vi "autonSample.vi"(0 "Auton Array":dbl[][](array[numeric]), 5 "MeasuredHeading":dbl, 9 "EncoderDistance":dbl) -> (4 "Left Drive":dbl(knob) scale=-1.0..1.0, 6 "Right Drive":dbl(knob) scale=-1.0..1.0, 10 "Turret Rotation":dbl, 14 "Feeder motor":dbl, 15 "Shooter motor output":dbl)   [LabVIEW 2011]
uses:
  Robot Global Data.vi
panel:
  out "Tzero":i64
  out "AccumDist":dbl
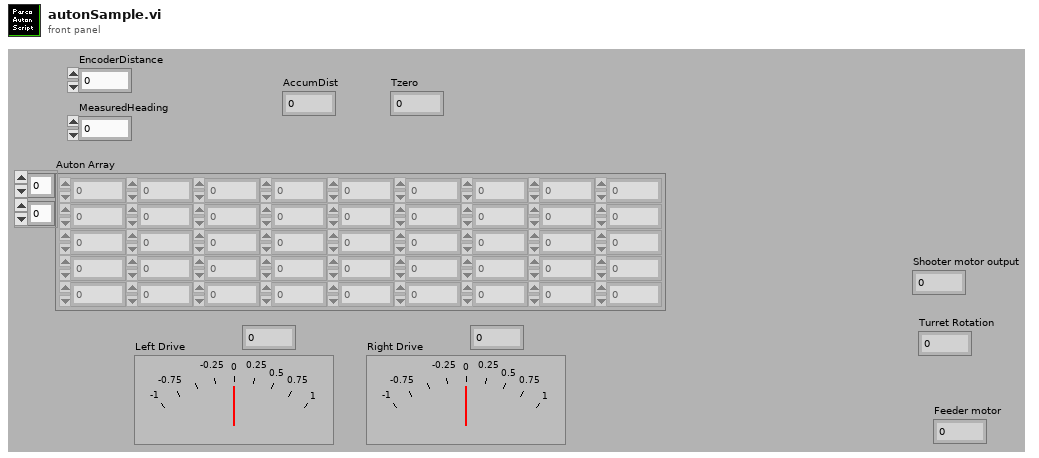
[diagram p1: front panel]
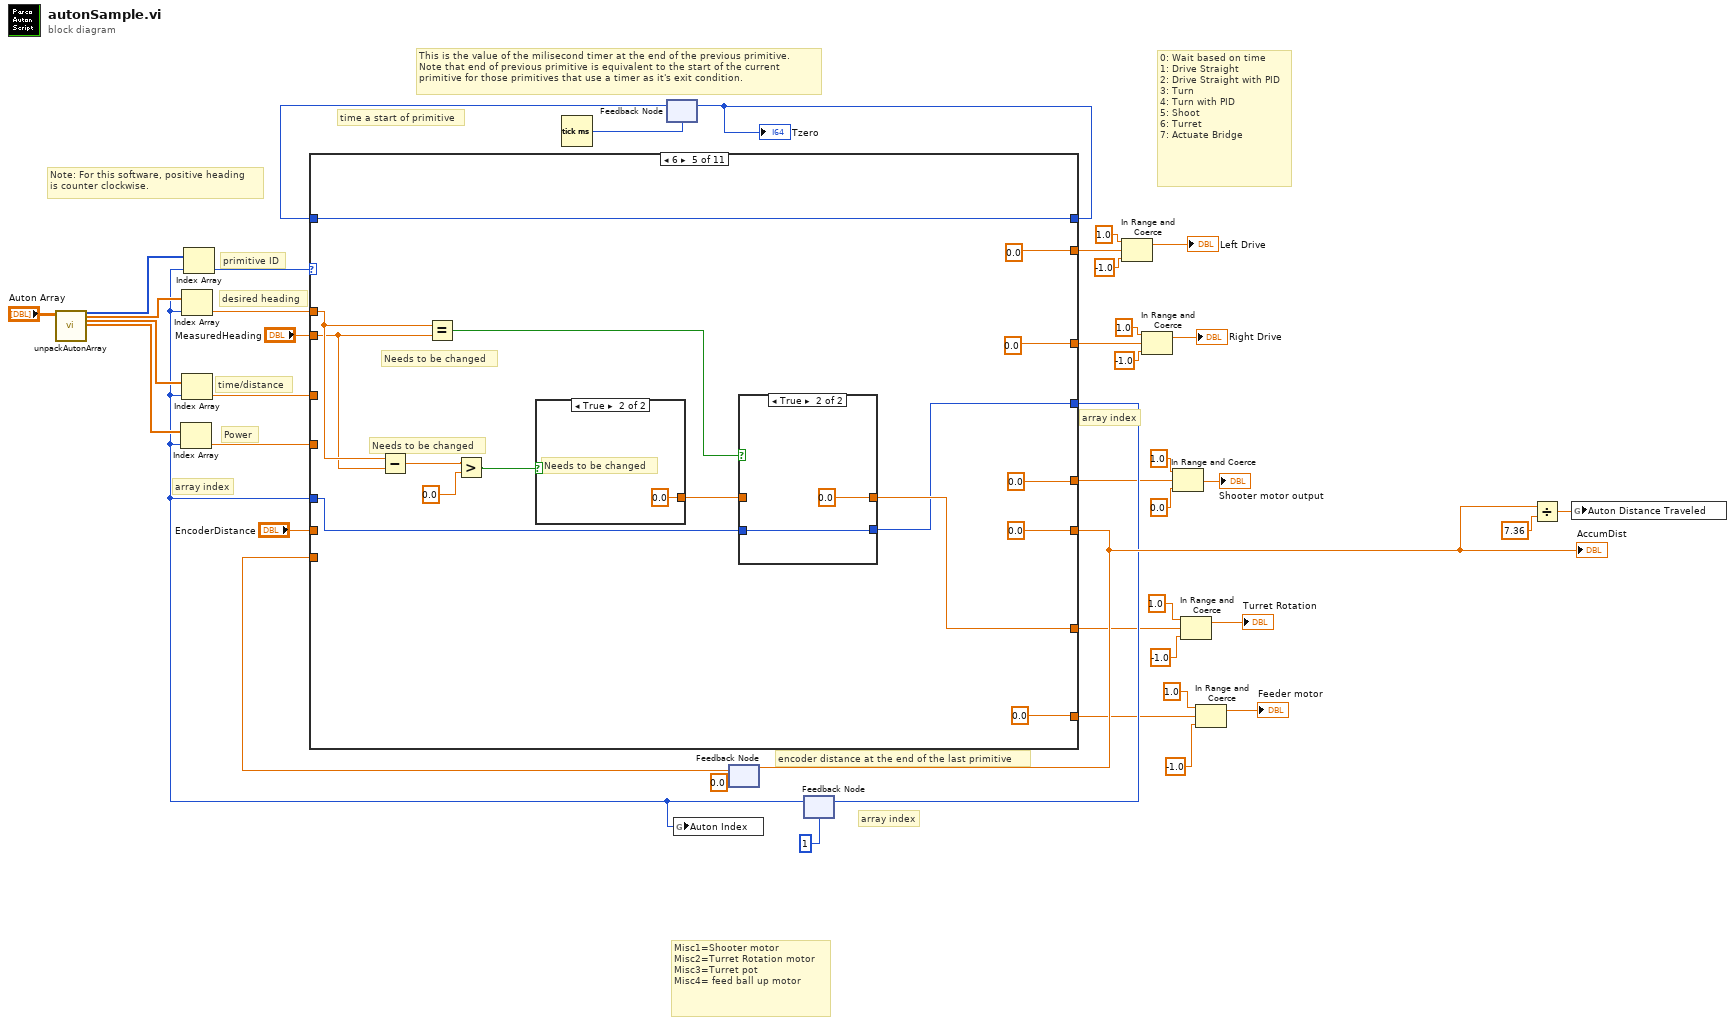
[diagram p0: block diagram]
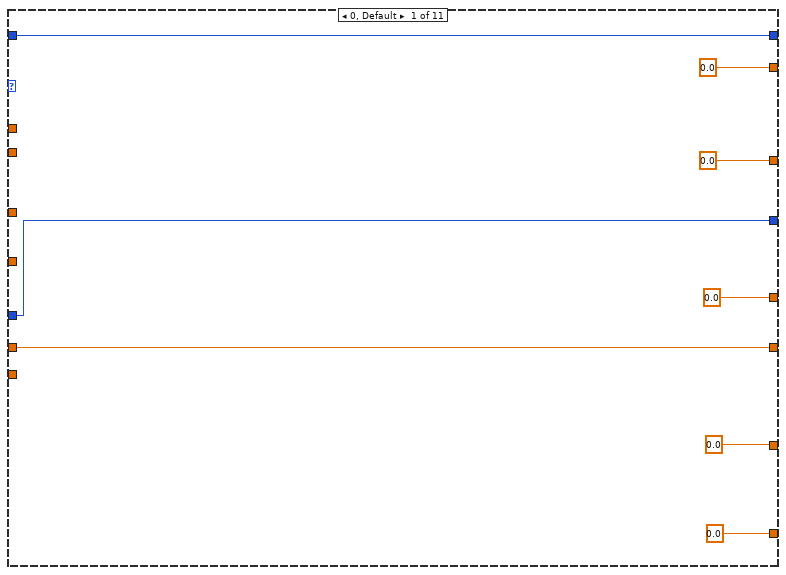
[diagram p2: hidden frame]
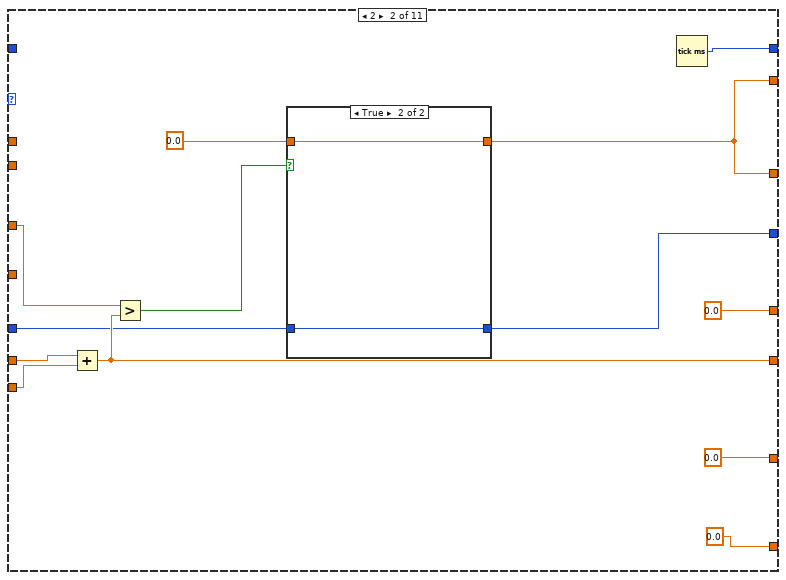
[diagram p3: hidden frame]
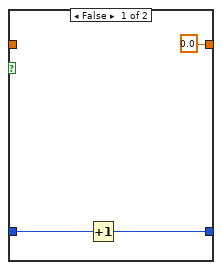
[diagram p4: hidden frame]
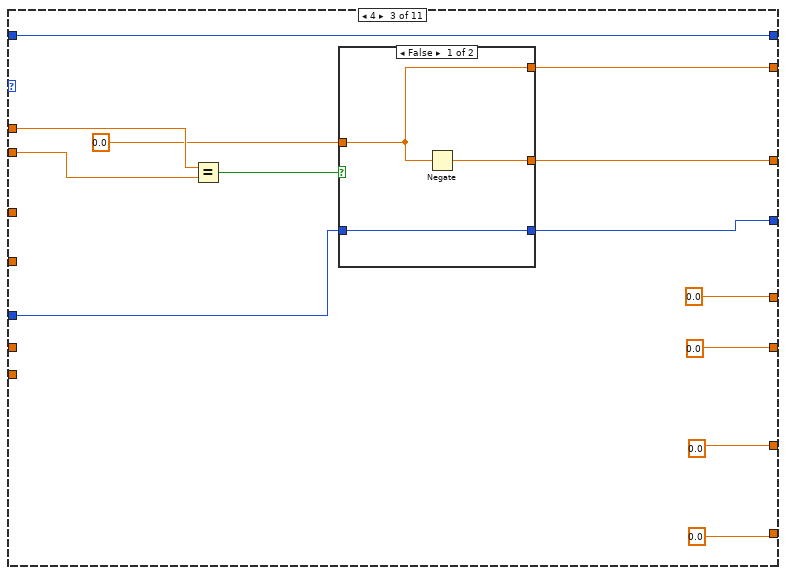
[diagram p5: hidden frame]
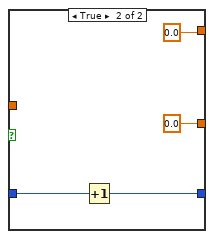
[diagram p6: hidden frame]
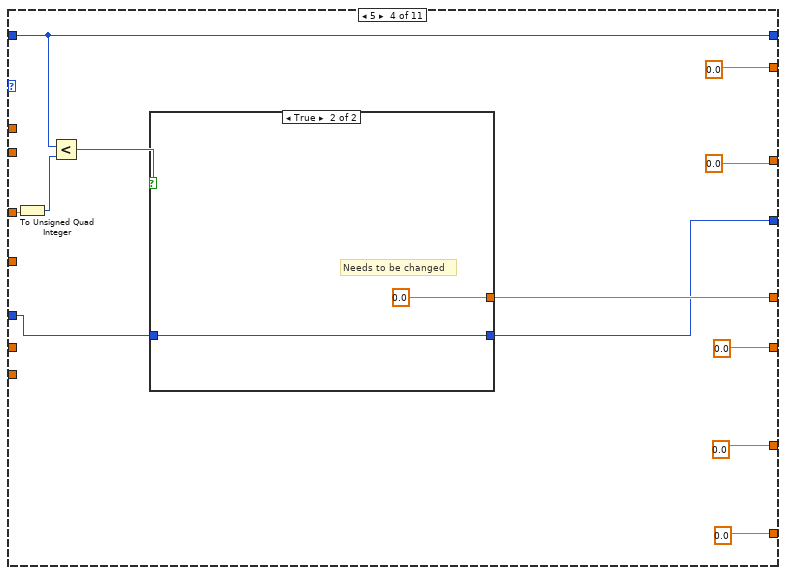
[diagram p7: hidden frame]
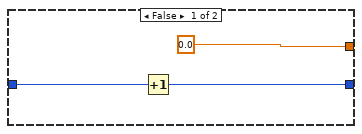
[diagram p8: hidden frame]
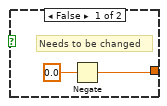
[diagram p10: hidden frame]
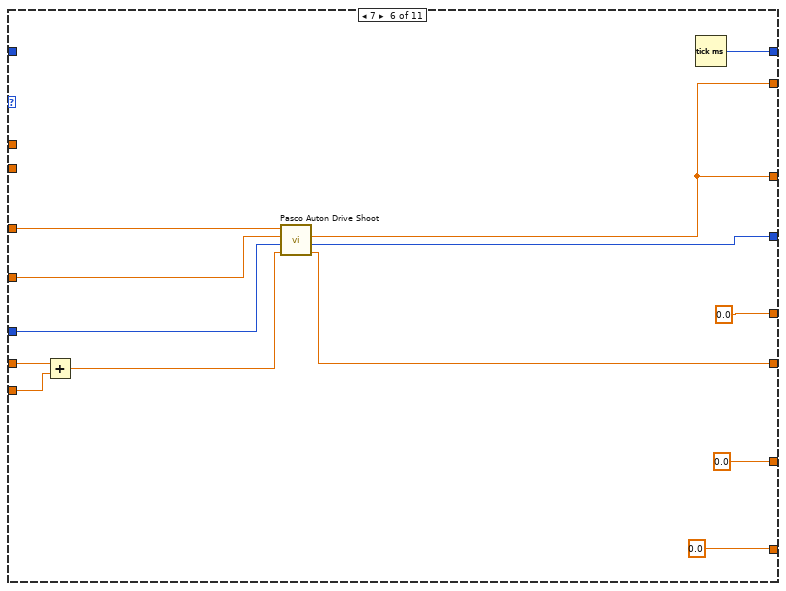
[diagram p11: hidden frame]
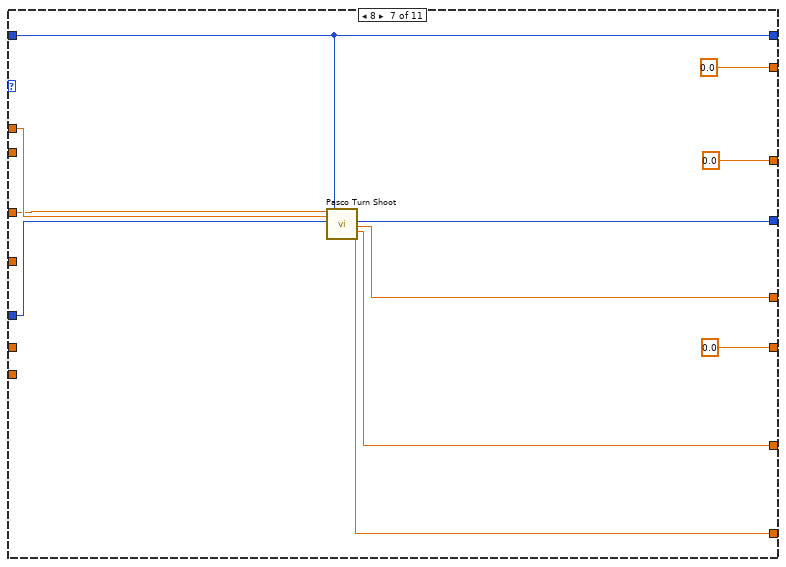
[diagram p12: hidden frame]
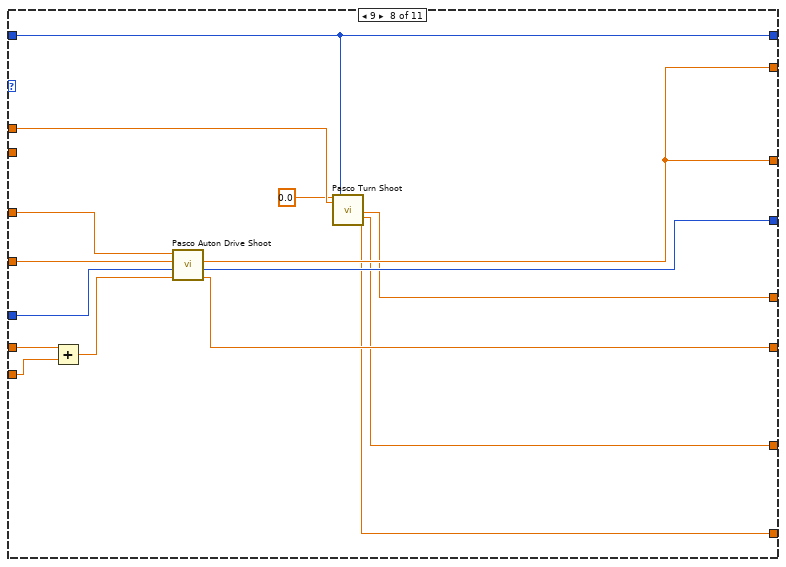
[diagram p13: hidden frame]
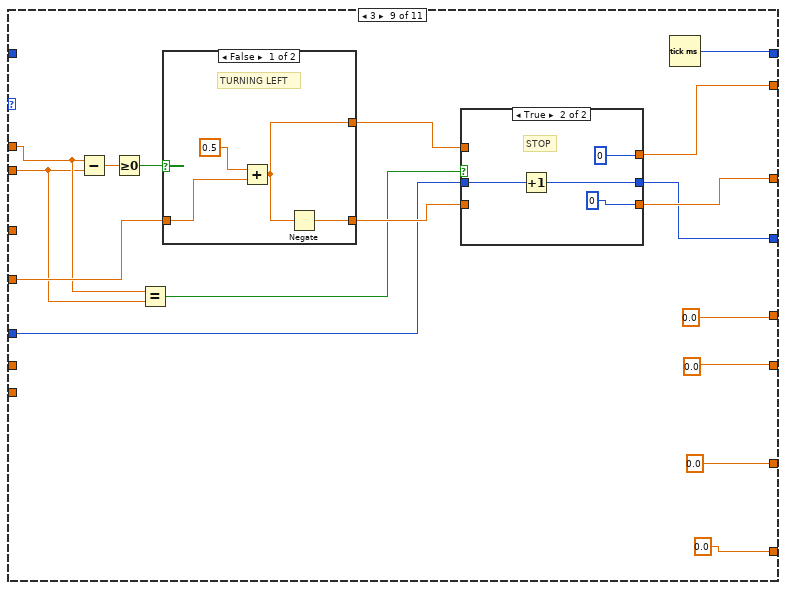
[diagram p14: hidden frame]
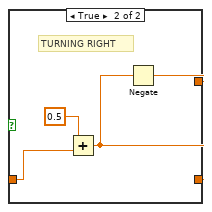
[diagram p16: hidden frame]
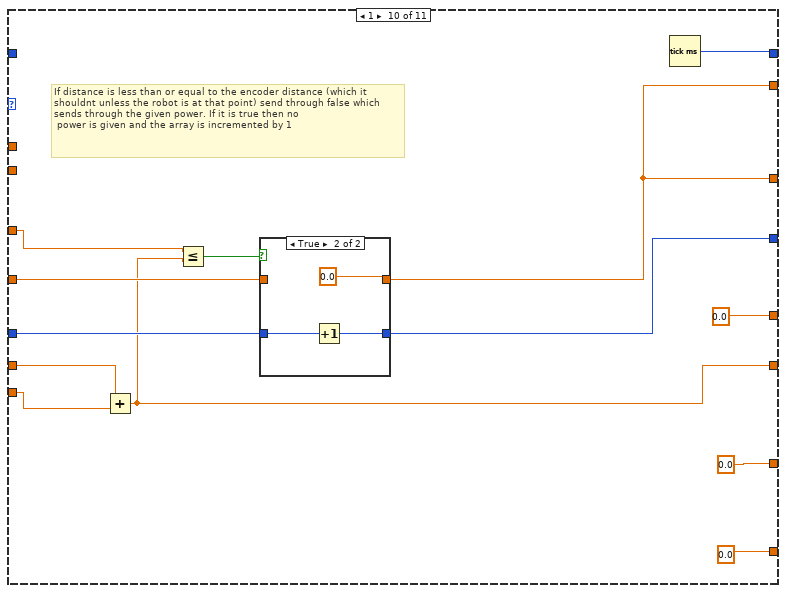
[diagram p17: hidden frame]
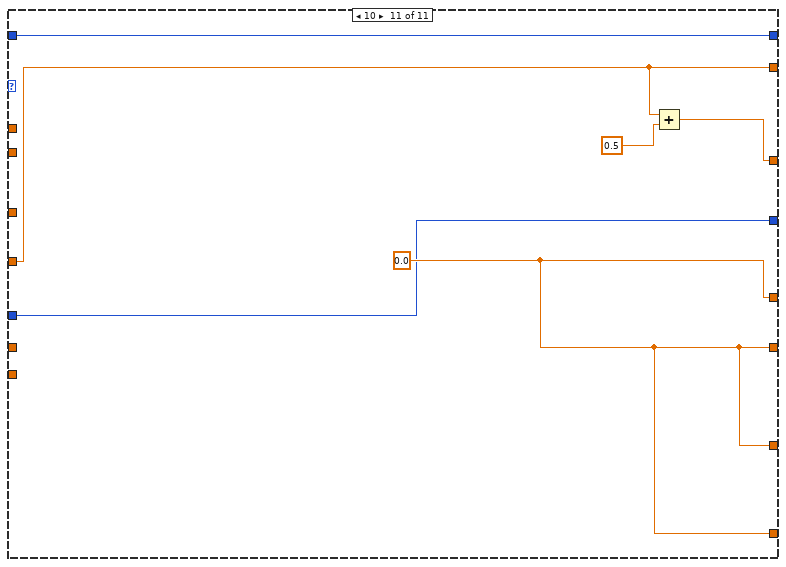
[diagram p19: hidden frame]
diagram:
  # "Misc1=Shooter motor\nMisc2=Turret Rotation motor\nMisc3=Turret pot\nMisc4= feed ball up motor"
  # "0: Wait based on time\n1: Drive Straight\n2: Drive Straight with PID\n3: Turn\n4: Turn with PID\n5: Shoot\n6: Turret\n7: Actuate Bridge"
  # "encoder distance at the end of the last primitive"
  # "Note: For this software, positive heading\nis counter clockwise."
  # "time a start of primitive"
  # "array index"
  # "array index"
  # "This is the value of the milisecond timer at the end of the previous primitive.\nNote that end of previous primitive is equivalent to the start of the current\nprimitive for those primitives that use a timer as it's exit condition."
  # "Power"
  # "array index"
  # "desired heading"
  # "primitive ID"
  # "time/distance"
  n1 = call "unpackAutonArray.vi"("all rows"="Auton Array") -> ("Primitive"=w41:i16[], "Heading"=w23:dbl[], "Distance/Time"=w24:dbl[], "Power"=w21:dbl[])  [unwired: 1 in, 22 out]
  n2 = Tick Count (ms)() -> (millisecond timer value=w35:u32)
  n3 = feedback #1(w35) -> (w39:u32)
  n4 = feedback #2(0.0 ("EncoderDistance")) -> (w20:dbl)
  n5 = feedback #3(1) -> (w2:i32)
  n6 = Index Array(array=w21, index=w2) -> (element=w37:dbl)
  n7 = Index Array(array=w23, index=w2) -> (element=w22:dbl)
  n8 = Index Array(array=w24, index=w2) -> (element=w38:dbl)
  n9 = Index Array(array=w41, index=w2) -> (element=w40:i16)
  n10 = case shown="6" w40 {
    tunnel: [w49 w55 w75 w95 w116 w134 w149 w160 w173 w206 w222] -> w15
    tunnel: w2 -> [w49 w56 w74 w96 w117 w137 w152 w165 w172 w207 w222]
    tunnel: [w46 w63 w81 w90 w115 w130 w150 w155 w179 w205 w221] -> w25
    tunnel: w39 -> [w46 _ w81 w90 w115 _ w150 w155 _ _ w221]
    tunnel: w38 -> [_ w59 _ w100 _ w141 w146 w167 _ w210 _]
    tunnel: w22 -> [_ _ w72 _ w121 _ w151 w159 w181 _ _]
    tunnel: [0.0 ("Current Setpoint") w57 w76 0.0 0.0 w135 0.0 w158 w175 w204 w219] -> w33
    tunnel: [0.0 ("Current Setpoint") w57 w77 0.0 0.0 w135 0.0 w158 w178 w204 w218] -> w26
    tunnel: w37 -> [_ _ _ _ _ w136 _ w166 w183 w208 w219]
    tunnel: "EncoderDistance" -> [w50 w62 _ _ _ w140 _ w164 _ w212 _]
    tunnel: "MeasuredHeading" -> [_ _ w71 _ w106 _ _ _ w180 _ _]
    tunnel: [w50 w60 0.0 0.0 0.0 w133 0.0 w161 0.0 w201 w223] -> w17
    tunnel: w20 -> [_ w61 _ _ _ w139 _ w163 _ w211 _]
    tunnel: [0.0 0.0 0.0 w97 0.0 0.0 ("Misc1  OUT") w148 w157 0.0 0.0 w223] -> w11
    tunnel: [0.0 0.0 0.0 0.0 w119 0.0 ("Misc1  OUT") w147 w156 0.0 0.0 w223] -> w7
    tunnel: [0.0 0.0 0.0 0.0 0.0 0.0 w142 w153 0.0 0.0 w223] -> w3
    frame 0, Default {
    }
    frame 2 {
      n11 = Add(x=w62, y=w61) -> (x+y=w60:dbl)
      n12 = Greater?(x=w59, y=w60) -> (0:w58:bool)
      n13 = case shown="True" w58 {
        tunnel: [0.0 w68] -> w57
        tunnel: 0.0 -> [_ w68]
        tunnel: w56 -> [w66 w67]
        tunnel: [w65 w67] -> w55
        frame False {
          n14 = Increment(x=w66) -> (x+1=w65:i32)
        }
        frame True {
        }
      }
      n15 = Tick Count (ms)() -> (millisecond timer value=w63:u32)
    }
    frame 4 {
      n16 = Equal?(x=w72, y=w71) -> (x = y?=w73:bool)
      n17 = case shown="False" w73 {
        tunnel: 0.0 ("output") -> [w83 _]
        tunnel: [w84 0.0] -> w77
        tunnel: [w83 0.0] -> w76
        tunnel: [w82 w87] -> w75
        tunnel: w74 -> [w82 w88]
        frame False {
          n18 = Negate(x=w83) -> (-x=w84:dbl)
        }
        frame True {
          n19 = Increment(x=w88) -> (x+1=w87:i32)
        }
      }
    }
    frame 5 {
      n20 = To Unsigned Quad Integer(1:w100) -> (0:w98:u64)
      n21 = Less?(x=w90, y=w98) -> (x < y?=w99:bool)
      n22 = case shown="True" w99 {
        tunnel: [0.0 0.0] -> w97
        tunnel: w96 -> [w102 w105]
        tunnel: [w101 w105] -> w95
        frame False {
          n23 = Increment(x=w102) -> (x+1=w101:i32)
        }
        frame True {
          # "Needs to be changed"
        }
      }
    }
    frame 6 {
      # "Needs to be changed"
      # "Needs to be changed"
      n24 = Subtract(x=w121, y=w106) -> (x-y=w108:dbl)
      n25 = Equal?(x=w121, y=w106) -> (x = y?=w120:bool)
      n26 = Greater?(x=w108, y=0.0) -> (0:w109:bool)
      n27 = case shown="True" w109 {
        tunnel: [w127 0.0] -> w118
        frame False {
          # "Needs to be changed"
          n28 = Negate(x=0.0) -> (-x=w127:dbl)
        }
        frame True {
          # "Needs to be changed"
        }
      }
      n29 = case shown="True" w120 {
        tunnel: [w123 0.0] -> w119
        tunnel: w118 -> [w123 _]
        tunnel: w117 -> [w122 w125]
        tunnel: [w122 w125] -> w116
        frame False {
        }
        frame True {
        }
      }
    }
    frame 7 {
      n30 = Add(x=w140, y=w139) -> (x+y=w138:dbl)
      n31 = call "Pasco Auton Drive Shoot.vi"("Encoder total"=w138, "Array"=w137, "Power"=w136, "time/distance"=w141) -> ("Encoder total"=w133:dbl, "Array Out"=w134:i32, "Power"=w135:dbl)  [unwired: 5 in]
      n32 = Tick Count (ms)() -> (millisecond timer value=w130:u32)
    }
    frame 8 {
      n33 = call "Pasco Turn Shoot.vi"("time/distance"=w146, "desired heading"=w151, "array index"=w152, "primitive time"=w150) -> ("array index"=w149:i32, "Misc1  OUT"=w148:dbl, "Misc2 OUT"=w147:dbl, "Misc4 OUT"=w142:dbl)  [unwired: 12 in]
    }
    frame 9 {
      n34 = Add(x=w164, y=w163) -> (x+y=w162:dbl)
      n35 = call "Pasco Auton Drive Shoot.vi"("Encoder total"=w162, "Array"=w165, "Power"=w166, "time/distance"=w167) -> ("Encoder total"=w161:dbl, "Array Out"=w160:i32, "Power"=w158:dbl)  [unwired: 5 in]
      n36 = call "Pasco Turn Shoot.vi"("time/distance"=0.0, "desired heading"=w159, "primitive time"=w155) -> ("Misc1  OUT"=w157:dbl, "Misc2 OUT"=w156:dbl, "Misc4 OUT"=w153:dbl)  [unwired: 13 in, 1 out]
    }
    frame 3 {
      n37 = Subtract(x=w181, y=w180) -> (x-y=w184:dbl)
      n38 = Greater Or Equal To 0?(x=w184) -> (x >= 0?=w182:bool)
      n39 = Equal?(x=w181, y=w180) -> (x = y?=w174:bool)
      n40 = case shown="False" w182 {
        tunnel: w183 -> [w194 w196]
        tunnel: [w192 w198] -> w176
        tunnel: [w193 w197] -> w177
        frame False {
          # "TURNING LEFT"
          n41 = Add(x=0.5, y=w194) -> (x+y=w192:dbl)
          n42 = Negate(x=w192) -> (-x=w193:dbl)
        }
        frame True {
          # "TURNING RIGHT"
          n43 = Add(x=0.5, y=w196) -> (x+y=w197:dbl)
          n44 = Negate(x=w197) -> (-x=w198:dbl)
        }
      }
      n45 = case shown="True" w174 {
        tunnel: w172 -> [w187 w191]
        tunnel: [w187 w190] -> w173
        tunnel: [w186 0] -> w178
        tunnel: w177 -> [w186 _]
        tunnel: [w185 0] -> w175
        tunnel: w176 -> [w185 _]
        frame False {
          # "DRIVE"
        }
        frame True {
          # "STOP"
          n46 = Increment(x=w191) -> (x+1=w190:i32)
        }
      }
      n47 = Tick Count (ms)() -> (millisecond timer value=w179:u32)
    }
    frame 1 {
      # "If distance is less than or equal to the encoder distance (which it shouldnt unless the robot is at that point) send through false which sends through the given power. If it is true then no\n power is given and the array is incremented by 1"
      n48 = Add(x=w212, y=w211) -> (x+y=w201:dbl)
      n49 = Less Or Equal?(x=w210, y=w201) -> (x <= y?=w209:bool)
      n50 = case shown="True" w209 {
        tunnel: [w214 0.0] -> w204
        tunnel: w208 -> [w214 _]
        tunnel: w207 -> [w213 w216]
        tunnel: [w213 w215] -> w206
        frame False {
        }
        frame True {
          n51 = Increment(x=w216) -> (x+1=w215:i32)
        }
      }
      n52 = Tick Count (ms)() -> (millisecond timer value=w205:u32)
    }
    frame 10 {
      w223 = 0.0
      n53 = Add(x=w219, y=0.5 ("x+y")) -> (x+y=w218:dbl)
    }
  }
  "AccumDist" <- w17
  "Tzero" <- w25
  n54 = feedback-in #1(w25) -> ()
  n55 = global write "Robot Global Data.vi" "Auton Index"(w2) -> ()
  n56 = feedback-in #2(w17) -> ()
  n57 = feedback-in #3(w15) -> ()
  n58 = In Range and Coerce(upper limit=1.0, x=w33, lower limit=-1.0) -> (coerced(x)=→"Left Drive":dbl)  [unwired: 1 out]
  n59 = In Range and Coerce(upper limit=1.0, x=w26, lower limit=-1.0) -> (coerced(x)=→"Right Drive":dbl)  [unwired: 1 out]
  n60 = In Range and Coerce(upper limit=1.0, x=w11, lower limit=0.0) -> (coerced(x)=→"Shooter motor output":dbl)  [unwired: 1 out]
  n61 = In Range and Coerce(upper limit=1.0, x=w7, lower limit=-1.0) -> (coerced(x)=→"Turret Rotation":dbl)  [unwired: 1 out]
  n62 = In Range and Coerce(upper limit=1.0, x=w3, lower limit=-1.0) -> (coerced(x)=→"Feeder motor":dbl)  [unwired: 1 out]
  n63 = Divide(x=w17, y=7.36) -> (x/y=w1:dbl)
  n64 = global write "Robot Global Data.vi" "Auton Distance Traveled"(w1) -> ()
